vi "Get Discovery Client.vi"(8 "error in (no error)":errorcluster, 11 "ClientPool in":refnum<class "GrpcClientPool.lvclass">) -> (0 "error out":errorcluster, 2 "Discovery grpc id":T1, 3 "ClientPool out":refnum<class "GrpcClientPool.lvclass">)   [LabVIEW 2020, in "gRPC Utilities.lvlib" / "GrpcClientPool.lvclass"]
uses:
  GrpcClientPool.lvclass
  <vilib>/gRPC/LabVIEW gRPC Library/Shared/grpcId.ctl
  GrpcClientPool.lvclass/GrpcClientPool.ctl
  <vilib>/gRPC/LabVIEW gRPC Library/grpc-lvsupport-release.lvlib
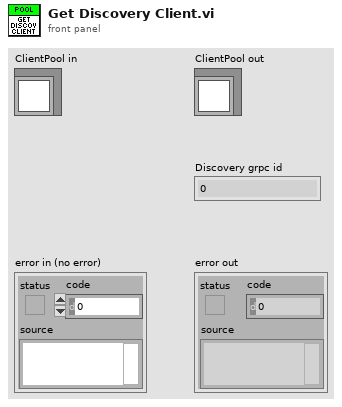
[diagram p1: front panel]
types:
  T1 = typedef "grpc-lvsupport-release.lvlib/grpcId.ctl" = u64
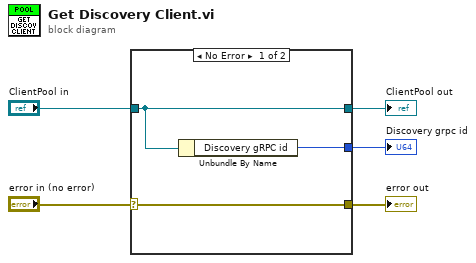
[diagram p0: block diagram]
diagram:
  n1 = case shown="No Error" "error in (no error)" {
    selector: "error in (no error)" -> [w7 w10]
    tunnel: [w7 w10] -> w4
    tunnel: [w8 w9] -> w2
    tunnel: "ClientPool in" -> [w8 w9]
    tunnel: [w6 _] -> w1
    frame No Error {
      n2 = Unbundle By Name(w8) -> ("Discovery gRPC id"=w6:T1)
    }
    frame Error {
    }
  }
  "error out" <- w4
  "ClientPool out" <- w2
  "Discovery grpc id" <- w1
